vi "ABB get temp rdgs.vi"(4 "Sim daq":bool, 6 "sim type":T1(ring), 7 "Simulate norma":bool, 8 "error in":errorcluster, 9 "# categories":i32, 10 "run config":T3, 11 "start":bool) -> (0 "error out":errorcluster, 1 "Category none rdgs":dbl[](array[numeric]), 2 "Measured temps":dbl[](array[numeric]), 3 "Category rdgs":dbl[](array[numeric]))   [LabVIEW 2017]
panel:
  out "Array 3":dbl[][](array[numeric])
  out "Numeric":i32
  out "Array":dbl[][](array[numeric])
  in  "Reading Category":T2(ring)=enum."Wdg Temp"
  in  "sim rise":dbl=50.0
  in  "sim time const":dbl=240.0
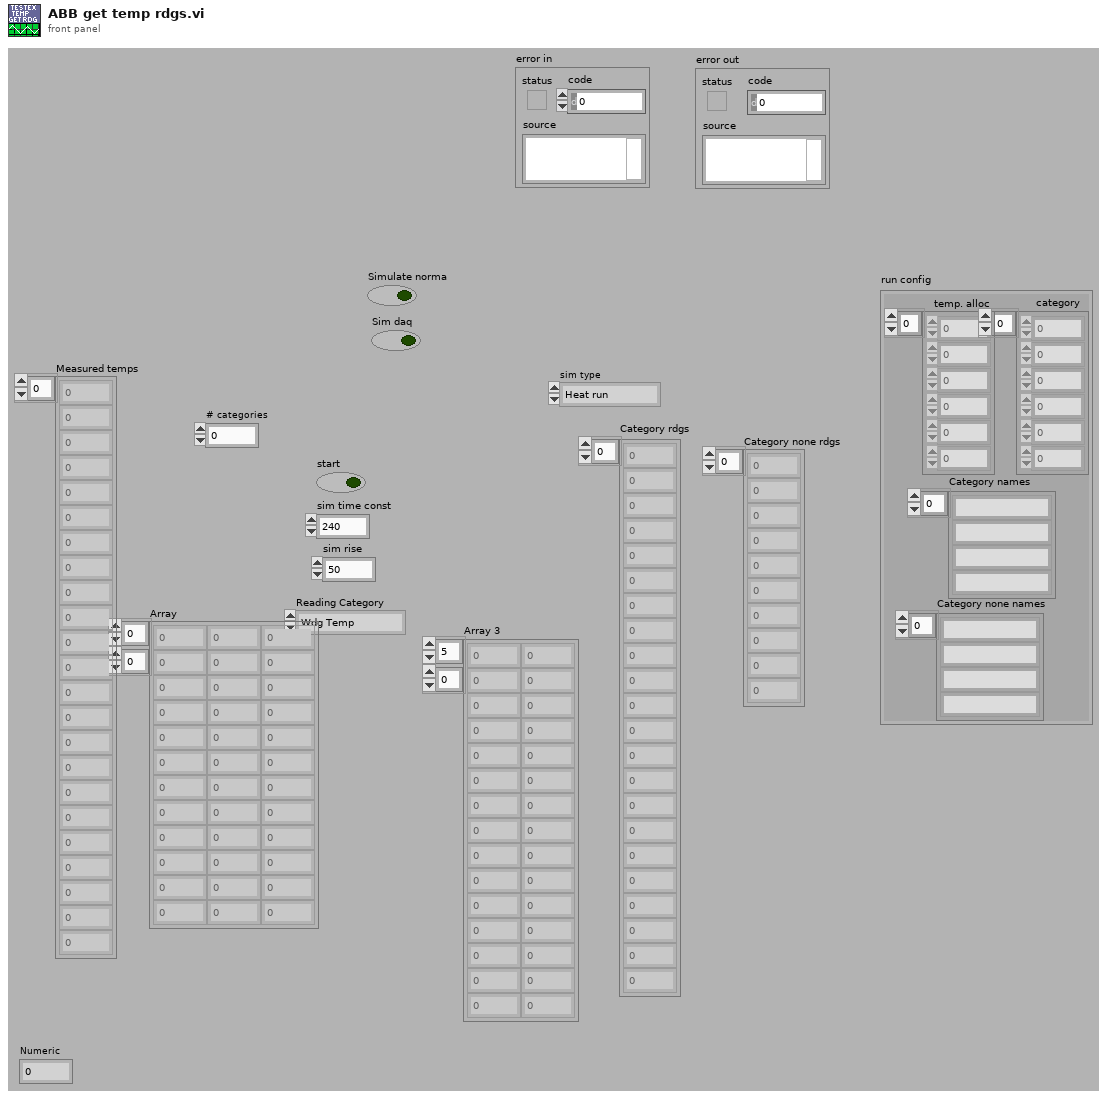
[diagram p1: front panel]
types:
  T1 = enum16{"Heat run", "Bearing run", "NoLd Heat Run", "Partial heat run"}
  T2 = enum16{"None", "Cool in", "Cool Out", "Wdg Temp", "Ambient", "DE", "NDE", "Aux coolant"}
  T3 = cluster{"temp. alloc":i32[], "category":i32[], "Category names":string[], "Category none names":string[]}
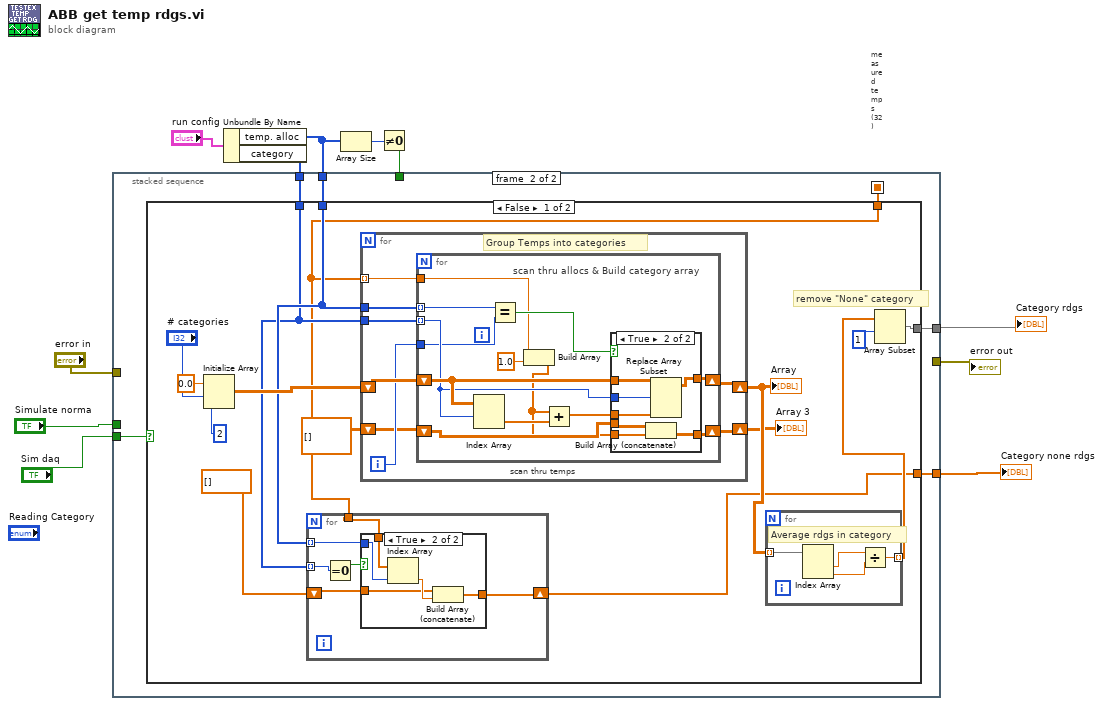
[diagram p0: block diagram]
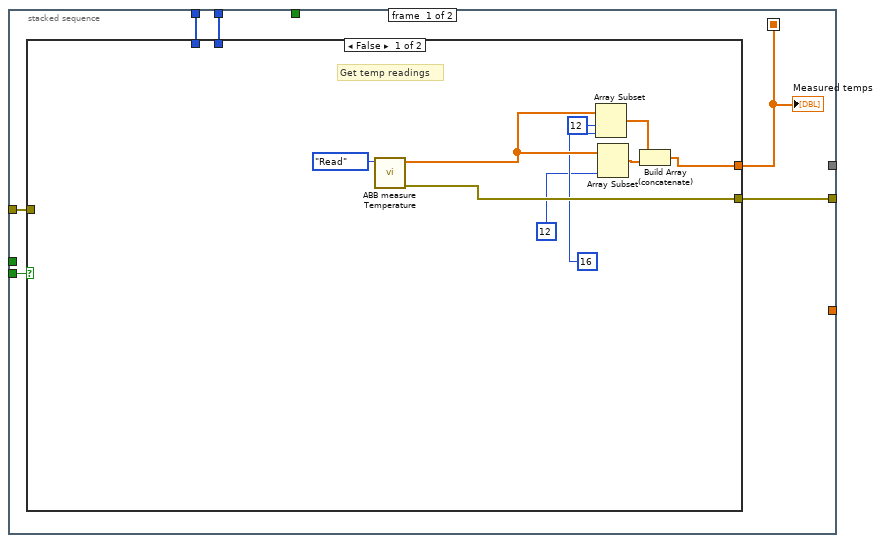
[diagram p2: hidden frame]
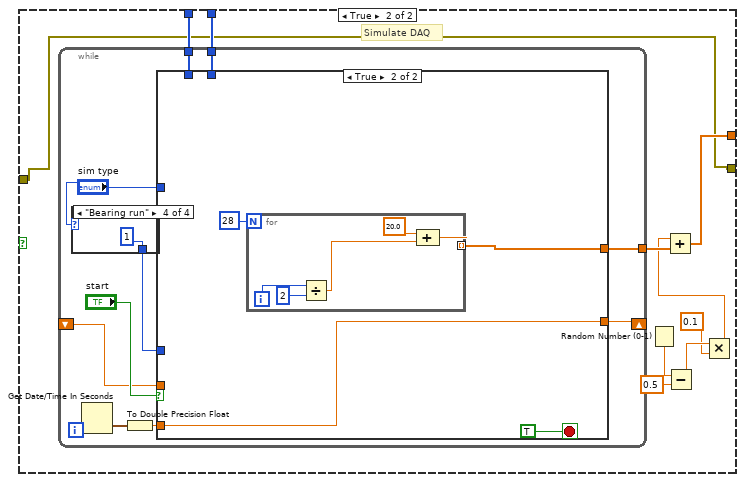
[diagram p3: hidden frame]
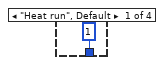
[diagram p4: hidden frame]
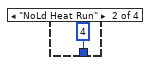
[diagram p5: hidden frame]
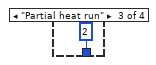
[diagram p6: hidden frame]
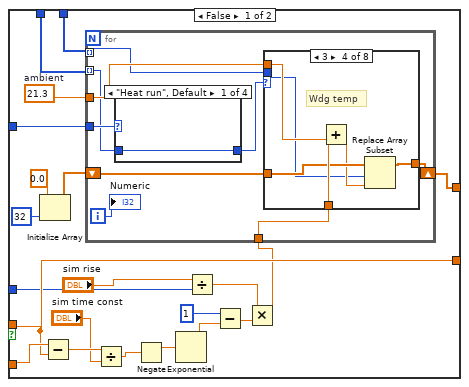
[diagram p7: hidden frame]
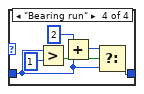
[diagram p10: hidden frame]
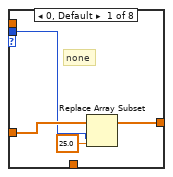
[diagram p11: hidden frame]
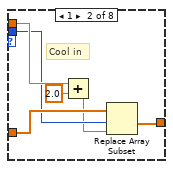
[diagram p12: hidden frame]
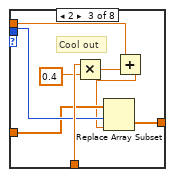
[diagram p13: hidden frame]
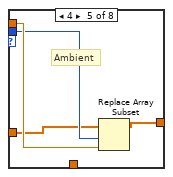
[diagram p14: hidden frame]
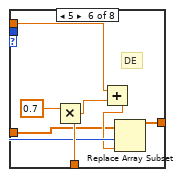
[diagram p15: hidden frame]
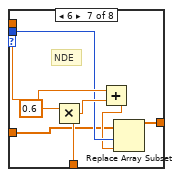
[diagram p16: hidden frame]
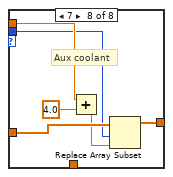
[diagram p17: hidden frame]
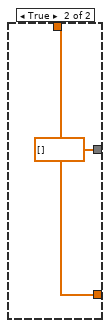
[diagram p20: hidden frame]
diagram:
  # "measured temps (32)"
  n1 = Unbundle By Name("run config") -> ("temp. alloc"=w4:i32[], "category"=w8:i32[])
  n2 = Array Size(array=w4) -> (size(s)=w3:i32)
  n3 = Not Equal To 0?(x=w3) -> (x != 0?=w2:bool)
  n4 = stacked-sequence {
    seq-local: [w13 _] -> [_ w151]
    tunnel: "Simulate norma" -> [_ _]
    tunnel: [_ w154] -> w10
    tunnel: w4 -> [w16 w153]
    tunnel: w8 -> [w17 w152]
    tunnel: [_ w150] -> w7
    tunnel: "error in" -> [w15 _]
    tunnel: [w14 _] -> w5
    tunnel: w2 -> [_ _]
    tunnel: "Sim daq" -> [w12 w149]
    frame #0 {
      n5 = case shown="False" w12 {
        tunnel: [w23 w29] -> w13
        tunnel: w17 -> [_ w35]
        tunnel: w16 -> [_ w34]
        tunnel: w15 -> [_ w27]
        tunnel: [w26 w27] -> w14
        frame False {
          # "Get temp readings"
          n6 = call "ABB measure Temperature.vi"("Mode"=enum16{"Initialise", "Read", "Close"}."Read") -> ("error out"=w26:errorcluster, "Readings"=w24:dbl[])  [unwired: 8 in, 1 out]
          n7 = Array Subset(array=w24, index=12, length=16) -> (w22:dbl[])
          n8 = Array Subset(array=w24, length=12 ("index")) -> (w21:dbl[])  [unwired: 1 in]
          n9 = Build Array (concatenate)(w22, w21) -> (w23:dbl[])
        }
        frame True {
          # "Simulate DAQ"
          n10 = while {
            tunnel: [w41] -> w36
            shift-right: [w42] -> _
            shift-left: _ -> [w45]
            tunnel: w35 -> [w40]
            tunnel: w34 -> [w39]
            stop <- TRUE stop-if-true
            n11 = case shown="\"Bearing run\"" "sim type" {
              tunnel: [1 4 2 1] -> w37
              frame "Heat run", Default {
              }
              frame "NoLd Heat Run" {
              }
              frame "Partial heat run" {
              }
              frame "Bearing run" {
              }
            }
            n12 = Get Date/Time In Seconds() -> (seconds since 1Jan1904=w44:timestamp)
            n13 = To Double Precision Float(number=w44) -> (double precision float=w43:dbl)
            n14 = case shown="True" "start" {
              tunnel: w45 -> [w63 _]
              tunnel: w43 -> [w72 w143]
              tunnel: [w63 w143] -> w42
              tunnel: [w55 w141] -> w41
              tunnel: w40 -> [w61 _]
              tunnel: w39 -> [w59 _]
              tunnel: "sim type" -> [w53 _]
              tunnel: w37 -> [w52 _]
              frame False {
                w60 = 21.3  # ambient
                n15 = Initialize Array(0.0, 32 ("dimension size")) -> (w56:dbl[])
                n16 = Subtract(x=w72, y=w63) -> (x-y=w71:dbl)
                n17 = Divide(x=w71, y="sim time const") -> (x/y=w69:dbl)
                n18 = Negate(x=w69) -> (-x=w68:dbl)
                n19 = Exponential(1:w68) -> (0:w66:dbl)
                n20 = Divide(x="sim rise", y=w52) -> (x/y=w54:dbl)
                n21 = Subtract(x=1, y=w66) -> (x-y=w65:dbl)
                n22 = Multiply(x=w54, y=w65) -> (x*y=w62:dbl)
                n23 = for {
                  tunnel: w61 -> [w74] mode=indexing
                  tunnel: w62 -> [w81]
                  tunnel: w60 -> [w80]
                  tunnel: w59 -> [w77] mode=indexing
                  shift-right: [w78] -> w55
                  shift-left: w56 -> [w79]
                  tunnel: w53 -> [w75]
                  i -> [w76]
                  n24 = case shown="\"Heat run\", Default" w75 {
                    tunnel: w74 -> [w82 w83 w84 w87]
                    tunnel: [w82 w83 w84 w88] -> w73
                    frame "Heat run", Default {
                    }
                    frame "NoLd Heat Run" {
                    }
                    frame "Partial heat run" {
                    }
                    frame "Bearing run" {
                      n25 = Greater?(x=w87, y=1) -> (0:w89:bool)
                      n26 = Add(x=2, y=w87) -> (x+y=w85:i32)
                      n27 = Select(t=w85, s=w89, f=w87) -> (s? t:f=w88:i32)
                    }
                  }
                  n28 = case shown="3" w73 {
                    tunnel: w81 -> [_ _ w108 w114 _ w125 w133 _]
                    tunnel: w80 -> [_ w100 w105 w113 w118 w126 w134 w140]
                    tunnel: w79 -> [w94 w98 w103 w112 w116 w119 w127 w137]
                    tunnel: [w93 w97 w102 w111 w115 w122 w130 w138] -> w78
                    tunnel: w77 -> [w92 w96 w104 w109 w117 w121 w129 w135]
                    frame 0, Default {
                      # "none"
                      n29 = Replace Array Subset(array=w94, new element=25.0 ("new element/subarray"), index=w92) -> (w93:dbl[])
                    }
                    frame 1 {
                      # "Cool in"
                      n30 = Add(x=w100, y=2.0) -> (x+y=w95:dbl)
                      n31 = Replace Array Subset(array=w98, new element=w95, index=w96) -> (w97:dbl[])
                    }
                    frame 2 {
                      # "Cool out"
                      n32 = Multiply(x=w108, y=0.4) -> (x*y=w106:dbl)
                      n33 = Add(x=w105, y=w106) -> (x+y=w101:dbl)
                      n34 = Replace Array Subset(array=w103, new element=w101, index=w104) -> (w102:dbl[])
                    }
                    frame 3 {
                      # "Wdg temp"
                      n35 = Add(x=w114, y=w113) -> (x+y=w110:dbl)
                      n36 = Replace Array Subset(array=w112, new element=w110, index=w109) -> (w111:dbl[])
                    }
                    frame 4 {
                      # "Ambient"
                      n37 = Replace Array Subset(array=w116, new element=w118, index=w117) -> (w115:dbl[])
                    }
                    frame 5 {
                      # "DE"
                      n38 = Multiply(x=0.7, y=w125) -> (x*y=w123:dbl)
                      n39 = Add(x=w126, y=w123) -> (x+y=w120:dbl)
                      n40 = Replace Array Subset(array=w119, new element=w120, index=w121) -> (w122:dbl[])
                    }
                    frame 6 {
                      # "NDE"
                      n41 = Multiply(x=0.6, y=w133) -> (x*y=w131:dbl)
                      n42 = Add(x=w134, y=w131) -> (x+y=w128:dbl)
                      n43 = Replace Array Subset(array=w127, new element=w128, index=w129) -> (w130:dbl[])
                    }
                    frame 7 {
                      # "Aux coolant"
                      n44 = Add(x=w140, y=4.0) -> (x+y=w136:dbl)
                      n45 = Replace Array Subset(array=w137, new element=w136, index=w135) -> (w138:dbl[])
                    }
                  }
                  "Numeric" <- w76
                }
              }
              frame True {
                n46 = for {
                  N: 28 -> [_]
                  tunnel: [w148] -> w141 mode=indexing
                  i -> [w147]
                  n47 = Divide(x=w147, y=2) -> (x/y=w144:dbl)
                  n48 = Compound Arithmetic op=ADD(20.0 ("y"), w144) -> (w148:dbl)
                }
              }
            }
          }
          n49 = Random Number (0-1)() -> (number: 0 to 1=w33:dbl)
          n50 = Subtract(x=w33, y=0.5) -> (x-y=w31:dbl)
          n51 = Multiply(x=w31, y=0.1) -> (x*y=w28:dbl)
          n52 = Add(x=w28, y=w36) -> (x+y=w29:dbl[])
        }
      }
      "Measured temps" <- w13
    }
    frame #1 {
      n53 = case shown="False" w149 {
        tunnel: [w164 dbl[] []] -> w154
        tunnel: w153 -> [w162 _]
        tunnel: w152 -> [w161 _]
        tunnel: w151 -> [w160 w217]
        tunnel: [w158 w217] -> w150
        frame False {
          # "remove \"None\" category"
          n54 = Initialize Array(0.0 ("element"), "# categories", 2) -> (w168:dbl[][])
          n55 = for {
            tunnel: w162 -> [w172] mode=indexing
            tunnel: w161 -> [w175] mode=indexing
            tunnel: w160 -> [w173]
            shift-right: [w171] -> w158
            shift-left: dbl[] [] -> [w170]
            n56 = Equal To 0?(x=w175) -> (x = 0?=w174:bool)
            n57 = case shown="True" w174 {
              tunnel: w173 -> [_ w181]
              tunnel: w172 -> [_ w180]
              tunnel: [w176 w178] -> w171
              tunnel: w170 -> [w176 w177]
              frame False {
              }
              frame True {
                n58 = Index Array(array=w181, index=w180) -> (element=w179:dbl)
                n59 = Build Array (concatenate)(w177, w179) -> (w178:dbl[])
              }
            }
          }
          n60 = for {
            tunnel: w161 -> [w190]
            tunnel: w160 -> [w193] mode=indexing
            tunnel: w162 -> [w192]
            shift-right: [w189] -> w166
            shift-left: w168 -> [w191]
            shift-right: [w187] -> w155
            shift-left: dbl[][] [] ("Array 3") -> [w186]
            i -> [w188]
            # "scan thru temps"
            # "Group Temps into categories"
            n61 = for {
              tunnel: w193 -> [w199]
              tunnel: w192 -> [w206] mode=indexing
              shift-right: [w203] -> w189
              shift-left: w191 -> [w204]
              tunnel: w190 -> [w200] mode=indexing
              tunnel: w188 -> [w198]
              shift-right: [w197] -> w187
              shift-left: w186 -> [w196]
              # "scan thru allocs & Build category array"
              n62 = Index Array(array=w204, index (row)=w200) -> (element=w195:dbl[])  [unwired: 1 in]
              n63 = Equal?(x=w206, y=w198) -> (x = y?=w201:bool)
              n64 = Build Array(w199, 1.0 ("element")) -> (w194:dbl[])
              n65 = Add(x=w194, y=w195) -> (x+y=w202:dbl[])
              n66 = case shown="True" w201 {
                tunnel: w204 -> [w208 w215]
                tunnel: [w208 w214] -> w203
                tunnel: w202 -> [_ w212]
                tunnel: w200 -> [_ w213]
                tunnel: [w207 w210] -> w197
                tunnel: w196 -> [w207 w211]
                tunnel: w194 -> [_ w209]
                frame False {
                }
                frame True {
                  n67 = Build Array (concatenate)(w211, w209) -> (w210:dbl[][])
                  n68 = Replace Array Subset(array=w215, new element=w212, index (row)=w213) -> (w214:dbl[][])  [unwired: 1 in]
                }
              }
            }
          }
          "Array" <- w166
          "Array 3" <- w155
          n69 = for {
            tunnel: w166 -> [w185] mode=indexing
            tunnel: [w182] -> w165 mode=indexing
            # "Average rdgs in category"
            n70 = Index Array(array=w185) -> (element #1=w184:dbl, element #2=w183:dbl)  [unwired: 2 in]
            n71 = Divide(x=w184, y=w183) -> (x/y=w182:dbl)
          }
          n72 = Array Subset(array=w165, index=1 ("length")) -> (w164:dbl[])  [unwired: 1 in]
        }
        frame True {
        }
      }
    }
  }
  "Category rdgs" <- w10
  "Category none rdgs" <- w7
  "error out" <- w5
